vi "Test.vi"(0 "Call Context":T8, 5 "Test Controls":T1 {"Slider" scale=-1.0..1.0}) -> (1 "SubState 0":T3=enum."driver control", 3 "Loop 0 Data":T5, 4 "SubState 1":T3, 6 "Loop 1 Data":T4, 10 "SubState 2":T3, 11 "SubState 3":T7, 15 "Loop 2 Data":T2)   [LabVIEW 2014]
uses:
  typedefs/state machine/singleUseSubstate.ctl
  typedefs/state machine/subStates.ctl
  typedefs/loop datatypes/Loop 2 Datatype.ctl
  typedefs/loop datatypes/Loop 1 Datatype.ctl
  typedefs/loop datatypes/Loop 0 Datatype.ctl
  global variables/state machine.vi
  typedefs/drive mode.ctl
  <vilib>/Rock Robotics/WPI/DriverStation/WPI_DriverStationDerivedRobotMode.ctl
  typedefs/test/test controls.ctl
panel:
  out "Compressor":bool
  out "JS Axis-Y 3":dbl
  out "JS Axis-X 3":dbl
  out "JS Axis-Y 2":dbl
  out "JS Axis-X 2":dbl
  out "UDB":bool
  out "JS Axis-X":dbl
  out "JS Axis-Y":dbl
  out "Exit Value":i32=-1
  # "Test Loop Data and Substates"
  # "Drive Loop"
  # "Loop 1: Lift"
  # "Loop 2: Container Arm"
  # "Loop 3: Tote Pistons"
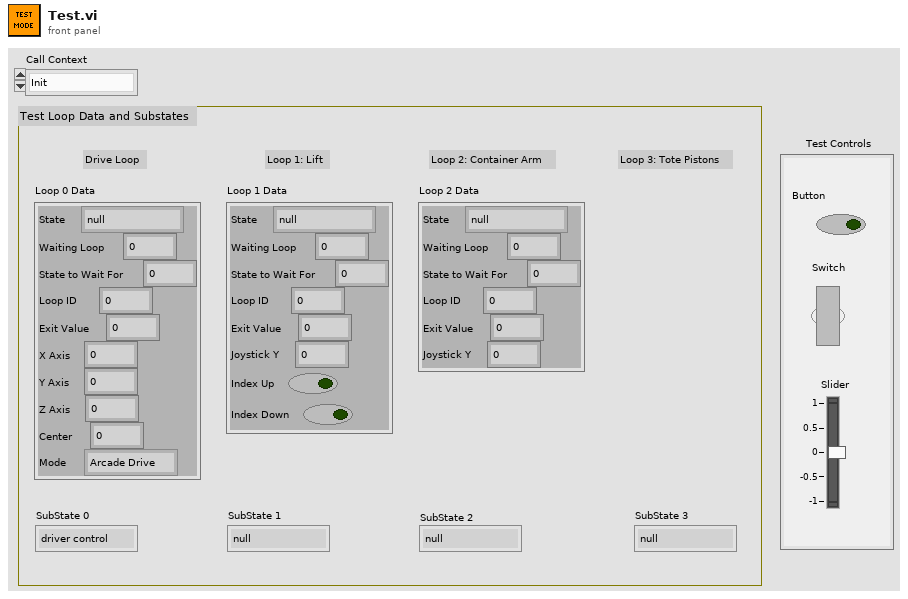
[diagram p1: front panel]
types:
  T1 = typedef "test controls.ctl" = cluster{"Button":bool, "Switch":bool, "Slider":dbl}
  T2 = typedef "Loop 2 Datatype.ctl" = cluster{"State":T3, "Waiting Loop":i32, "State to Wait For":i32, "Loop ID":i32, "Exit Value":i32, "Joystick Y":dbl}
  T3 = typedef "subStates.ctl" = enum16{"null", "wait", "driver control", "auto", "manual override", "hold position", "rotate", "test", "end"}
  T4 = typedef "Loop 1 Datatype.ctl" = cluster{"State":T3, "Waiting Loop":i32, "State to Wait For":i32, "Loop ID":i32, "Exit Value":i32, "Joystick Y":dbl, "Index Up":bool, "Index Down":bool}
  T5 = typedef "Loop 0 Datatype.ctl" = cluster{"State":T3, "Waiting Loop":i32, "State to Wait For":i32, "Loop ID":i32, "Exit Value":i32, "X Axis":dbl, "Y Axis":dbl, "Z Axis":dbl, "Center":dbl, "Mode":T6}
  T6 = typedef "drive mode.ctl" = enum16{"Arcade Drive", "H-Drive", "H-Drive PID"}
  T7 = typedef "singleUseSubstate.ctl" = enum16{"null", "wait", "extend left", "retract left", "extend right", "retract right", "end"}
  T8 = typedef "WPI_DriverStationDerivedRobotMode.ctl" = enum16{"Init", "Execute", "Stop"}
  T9 = typedef "WPI_JoystickDevRef.ctl" = cluster{"Device":T10}
  T10 = typedef "WPI_JoystickDeviceEnum.ctl" = enum16{"USB 0", "USB 1", "USB 2", "USB 3", "USB 4", "USB 5"}
  T11 = typedef "singleUseSubstate.ctl" = enum16{"null", "wait", "extend", "retract", "end"}
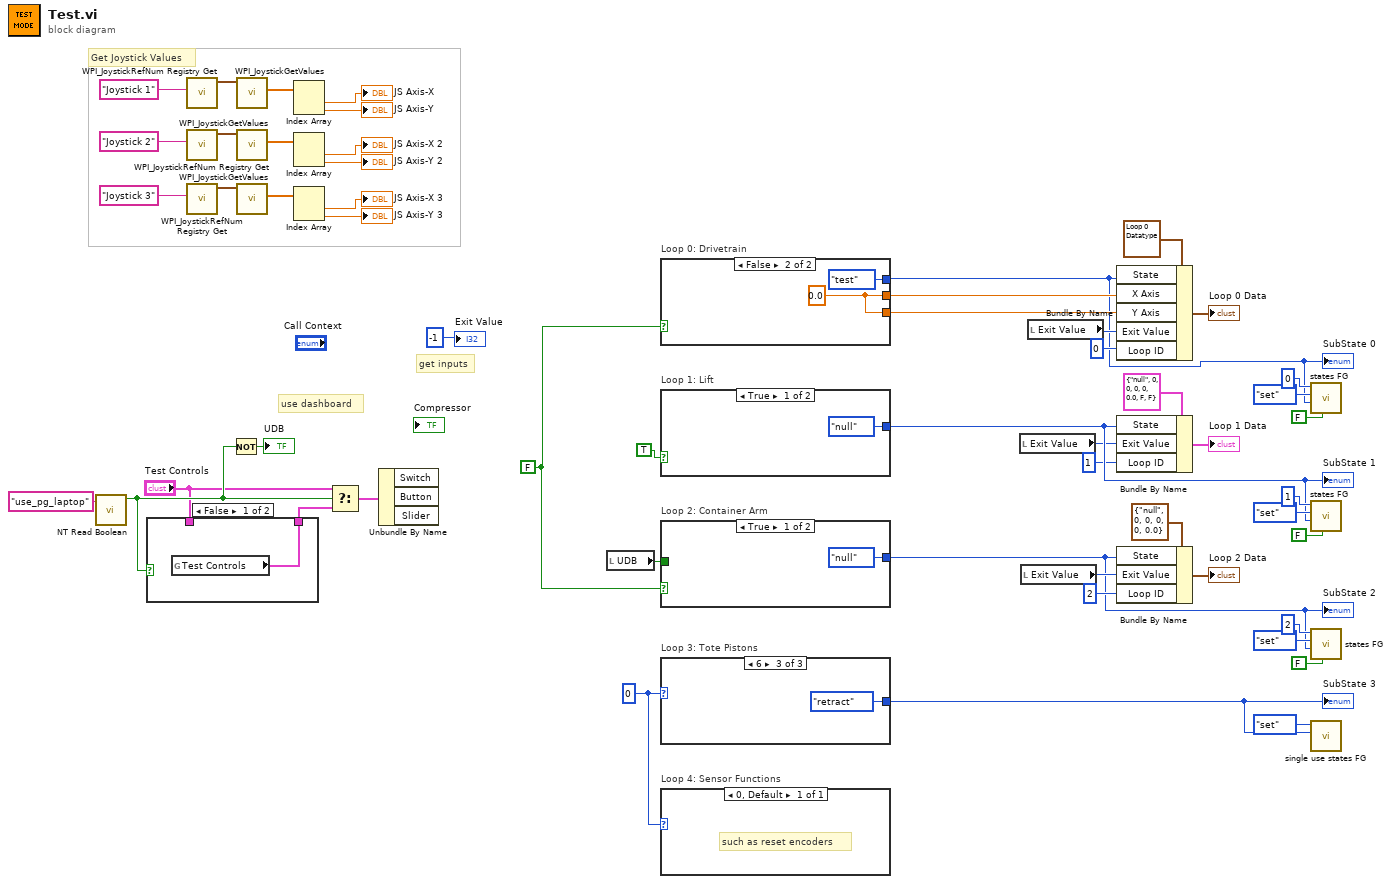
[diagram p0: block diagram]
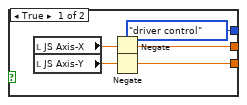
[diagram p3: hidden frame]
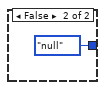
[diagram p4: hidden frame]
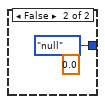
[diagram p5: hidden frame]
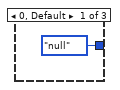
[diagram p6: hidden frame]
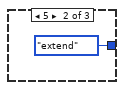
[diagram p7: hidden frame]
diagram:
  w15 = 0 ("Button Pressed")
  w18 = FALSE
  # "use dashboard"
  # "get inputs"
  # "Get Joystick Values"
  n1 = call <vilib>:"NT Read Boolean.vi"("Name"="use_pg_laptop") -> ("Boolean"=w28:bool)  [unwired: 9 in, 1 out]
  n2 = case shown="False" w28 {
    tunnel: [w55 w56] -> w26
    tunnel: "Test Controls" -> [_ w56]
    frame False {
      n3 = global read "state machine.vi" "Test Controls"() -> (w55:T1)
    }
    frame True {
    }
  }
  n4 = call <vilib>:"WPI_JoystickRefNum Registry Get.vi"("refnum name"="Joystick 1") -> ("JoystickDevRef"=w52:T9)  [unwired: 9 in, 1 out]
  n5 = call <vilib>:"WPI_JoystickRefNum Registry Get.vi"("refnum name"="Joystick 2") -> ("JoystickDevRef"=w25:T9)  [unwired: 9 in, 1 out]
  n6 = call <vilib>:"WPI_JoystickRefNum Registry Get.vi"("refnum name"="Joystick 3") -> ("JoystickDevRef"=w22:T9)  [unwired: 9 in, 1 out]
  n7 = Not(x=w28) -> (.not. x?=→"UDB":bool)
  n8 = call <vilib>:"WPI_JoystickGetValues.vi"("JoystickDevRef"=w52) -> ("Axes"=w14:dbl[])  [unwired: 6 in, 4 out]
  n9 = call <vilib>:"WPI_JoystickGetValues.vi"("JoystickDevRef"=w25) -> ("Axes"=w13:dbl[])  [unwired: 6 in, 4 out]
  n10 = call <vilib>:"WPI_JoystickGetValues.vi"("JoystickDevRef"=w22) -> ("Axes"=w12:dbl[])  [unwired: 6 in, 4 out]
  n11 = Index Array(array=w14) -> (element #1=→"JS Axis-X":dbl, element #2=→"JS Axis-Y":dbl)  [unwired: 2 in]
  n12 = Index Array(array=w13) -> (element #1=→"JS Axis-X 2":dbl, element #2=→"JS Axis-Y 2":dbl)  [unwired: 2 in]
  n13 = Index Array(array=w12) -> (element #1=→"JS Axis-X 3":dbl, element #2=→"JS Axis-Y 3":dbl)  [unwired: 2 in]
  n14 = Select(t="Test Controls", s=w28, f=w26) -> (s? t:f=w29:T1)
  n15 = Unbundle By Name(w29) -> ()  [unwired: 3 out]
  n16 = local read "UDB"() -> (w20:bool)
  n17 = case "Loop 0: Drivetrain" shown="False" w18 {
    tunnel: [w57 w62] -> w31
    tunnel: [subStates."driver control" ("State") subStates."test" ("State")] -> w1
    tunnel: [w58 w62] -> w32
    frame True {
      n18 = local read "JS Axis-X"() -> (w60:dbl)
      n19 = local read "JS Axis-Y"() -> (w59:dbl)
      n20 = Negate(x=w60) -> (-x=w58:dbl)
      n21 = Negate(x=w59) -> (-x=w57:dbl)
    }
    frame False {
      w62 = 0.0 ("JS Axis-X")
    }
  }
  "SubState 0" <- w1
  n22 = case "Loop 1: Lift" shown="True" TRUE {
    tunnel: [subStates."null" ("State") subStates."null" ("State")] -> w39
    frame True {
    }
    frame False {
    }
  }
  "SubState 1" <- w39
  n23 = case "Loop 2: Container Arm" shown="True" w18 {
    tunnel: [subStates."null" ("State") subStates."null" ("State")] -> w19
    tunnel: w20 -> [_ _]
    frame True {
    }
    frame False {
      (unwired) 0.0 ("Belts")
    }
  }
  "SubState 2" <- w19
  n24 = case "Loop 3: Tote Pistons" shown="6" w15 {
    tunnel: [singleUseSubstate."null" ("SubState 4") singleUseSubstate."extend" ("SubState 4") singleUseSubstate."retract" ("SubState 4")] -> w5
    frame 0, Default {
    }
    frame 5 {
    }
    frame 6 {
    }
  }
  "SubState 3" <- w5
  n25 = case "Loop 4: Sensor Functions" shown="0, Default" w15 {
    frame 0, Default {
      # "such as reset encoders"
    }
  }
  n26 = local read "Exit Value"() -> (w3:i32)
  n27 = local read "Exit Value"() -> (w48:i32)
  n28 = local read "Exit Value"() -> (w36:i32)
  n29 = Bundle By Name(cluster=T5 {"State"=enum."null", "Waiting Loop"=0, "State to Wait For"=0, "Loop ID"=0, "Exit Value"=0, "X Axis"=0.0, "Y Axis"=0.0, "Z Axis"=0.0, "Center"=0.0, "Mode"=enum."Arcade Drive"} ("Loop 0 Data"), "State"=w1, "X Axis"=w32, "Y Axis"=w31, "Exit Value"=w36, "Loop ID"=0) -> (→"Loop 0 Data":T5)
  n30 = Bundle By Name(cluster=T4 {"State"=enum."null", "Waiting Loop"=0, "State to Wait For"=0, "Loop ID"=0, "Exit Value"=0, "Joystick Y"=0.0, "Index Up"=FALSE, "Index Down"=FALSE} ("Loop 1 Data"), "State"=w39, "Exit Value"=w3, "Loop ID"=1) -> (→"Loop 1 Data":T4)
  n31 = Bundle By Name(cluster=T2 {"State"=enum."null", "Waiting Loop"=0, "State to Wait For"=0, "Loop ID"=0, "Exit Value"=0, "Joystick Y"=0.0} ("Loop 2 Data"), "State"=w19, "Exit Value"=w48, "Loop ID"=2) -> (→"Loop 2 Data":T2)
  n32 = call "states FG.vi"("exit in"=FALSE, "subState in"=w1, "menu (get)"=enum16{"set", "get"}."set", "Loop ID"=0) -> ()  [unwired: 4 in, 4 out]
  n33 = call "states FG.vi"("exit in"=FALSE, "subState in"=w39, "menu (get)"=enum16{"set", "get"}."set", "Loop ID"=1) -> ()  [unwired: 4 in, 4 out]
  n34 = call "states FG.vi"("exit in"=FALSE, "subState in"=w19, "menu (get)"=enum16{"set", "get"}."set", "Loop ID"=2) -> ()  [unwired: 4 in, 4 out]
  n35 = call "single use states FG.vi"("substate"=w5, "menu (get)"=enum16{"set", "get"}."set") -> ()  [unwired: 6 in, 4 out]
  "Exit Value" <- -1 ("Exit Value")
